vi "Read_CubeLiftOutput.vi"(8 "error in (no error)":errorcluster, 11 "CubeLiftData in":refnum<class "CubeLiftData.lvclass">) -> (0 "error out":errorcluster, 2 "CubeLiftOutput":T1 {"LiftControlMode" items=["PercentOutput"=0, "Position"=1, "Velocity"=2, "Current"=3, "Follower"=5, "MotionProfile"=6, "MotionMagic"=7, "MotionMagicArc"=8, "MotionProfileArc"=10, "Disabled"=15]}, 3 "CubeLiftData out":refnum<class "CubeLiftData.lvclass">)   [LabVIEW 2017, in "CubeLiftData.lvclass"]
uses:
  CubeLiftData.lvclass
  Team-code/CubeLiftOutput.ctl
  <vilib>/Rock Robotics/WPI/ThirdParty/Phoenix-LabVIEW/Motor Controller/Controls/CTRE_Phoenix_MotorControl_ControlMode.ctl
  CubeLiftData.lvclass/CubeLiftData.ctl
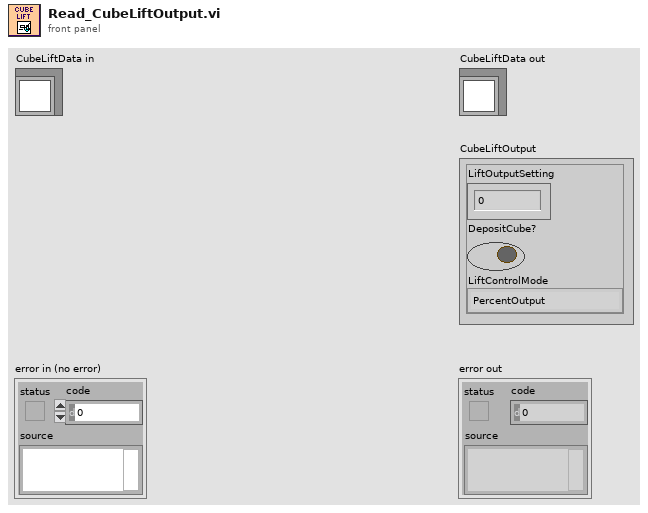
[diagram p1: front panel]
types:
  T1 = typedef "CubeLiftData.lvclass/CubeLiftOutput.ctl" = cluster{"LiftOutputSetting":dbl, "DepositCube?":bool, "LiftControlMode":T2}
  T2 = typedef "CTRE_Phoenix_MotorControl_ControlMode.ctl" = u16
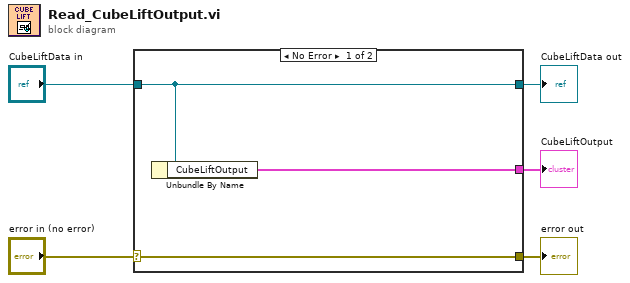
[diagram p0: block diagram]
diagram:
  n1 = case shown="No Error" "error in (no error)" {
    selector: "error in (no error)" -> [w8 w9]
    tunnel: [w8 w9] -> w4
    tunnel: [w7 w10] -> w2
    tunnel: "CubeLiftData in" -> [w7 w10]
    tunnel: [w6 _] -> w1
    frame No Error {
      n2 = Unbundle By Name(w7) -> ("CubeLiftOutput"=w6:T1)
    }
    frame Error {
    }
  }
  "error out" <- w4
  "CubeLiftData out" <- w2
  "CubeLiftOutput" <- w1
